vi "Select OPC Tags.vi"(7 "Mode":T1, 8 "error in":errorcluster, 11 "Section Ptr":T2 format="%.0x") -> (0 "error out":errorcluster)   [LabVIEW 2013, in "OPC UA Client System Explorer.lvlib"]
uses:
  OPC UA Client System Explorer.lvlib
  <vilib>/NI Veristand/Custom Device API/Custom Device Item Ref.ctl
  Types/Tag Selection Mode.ctl
  <vilib>/NI/AMC/Read Termination Message.vi
  <vilib>/NI/AMC/Create Single Message.vi
  <vilib>/NI/AMC/Update Message Routing Info.vi
  <vilib>/NI/AMC/Create Multiple Messages.vi
  <vilib>/NI/AMC/Globals.vi
  <vilib>/NI/AMC/Send Message.vi
  <vilib>/NI/AMC/AMC.lvlib
  <vilib>/NI Veristand/Custom Device API/Custom Device API.lvlib
panel:
  in  "OK":bool
  in  "Cancel":bool
  in  "Tree":string(tree)
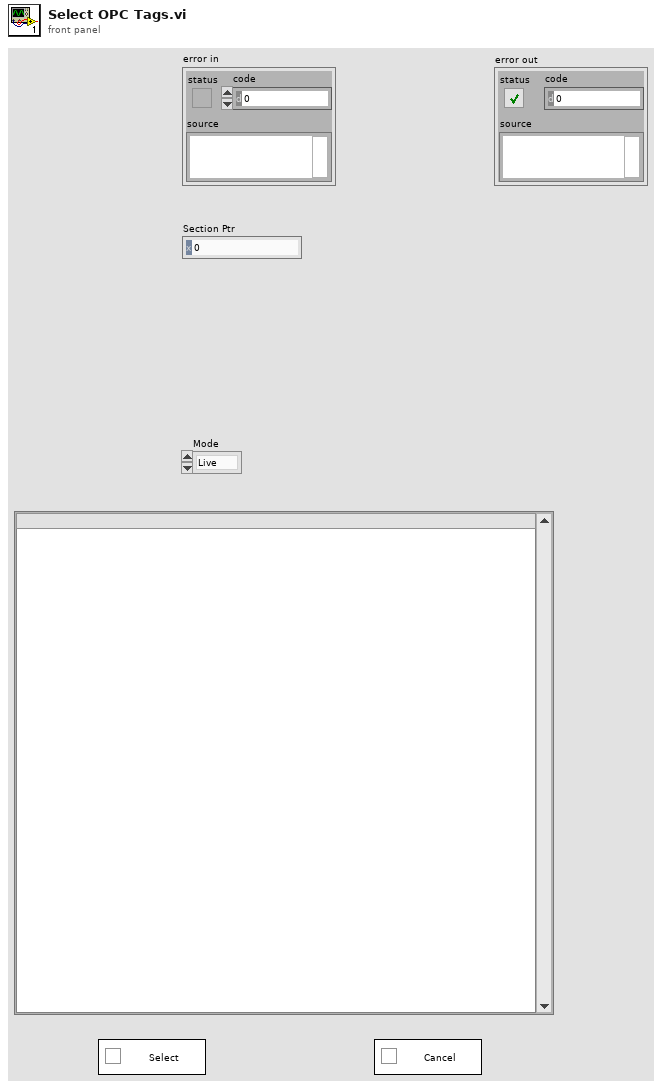
[diagram p1: front panel]
types:
  T1 = typedef "OPC UA Client System Explorer.lvlib/Tag Selection Mode.ctl" = enum8{"Live", "Offline"}
  T2 = typedef "Custom Device API.lvlib/Custom Device Item Ref.ctl" = u64
  T3 = cluster{"name":string, "node type":enum32{"Other", "Folder", "Item/Property"}, "DataType":u32, "access":enum16{"Null", "Read", "Write", "Read&Write"}, "description":string}
  T4 = typedef "AMC.lvlib/Message Queue.ctl" = refnum<queue>
  T5 = typedef "Custom Device API.lvlib/Custom Device Item Info.ctl" = cluster{"Name":string, "Is Channel":bool, "GUID":string, "Is Waveform":bool}
  T6 = typedef "OPC UA Client Shared.lvlib/Connection.Properties.ctl" = cluster{"Server IP Address":string, "Server Port":u16, "Message Mode":enum16{"None", "Sign", "Sign and Encrypt"}, "Security":enum16{"Basic256", "Basic128Rsa15"}, "User Name":string, "Password":string, "Client Certificate":path, "Server Certificate":path, "Server Certificate (RT)":path, "Client Certificate (RT)":path}
  T7 = typedef "LVPoint32TypeDef.ctl" = cluster{"Horizontal":i32, "Vertical":i32}
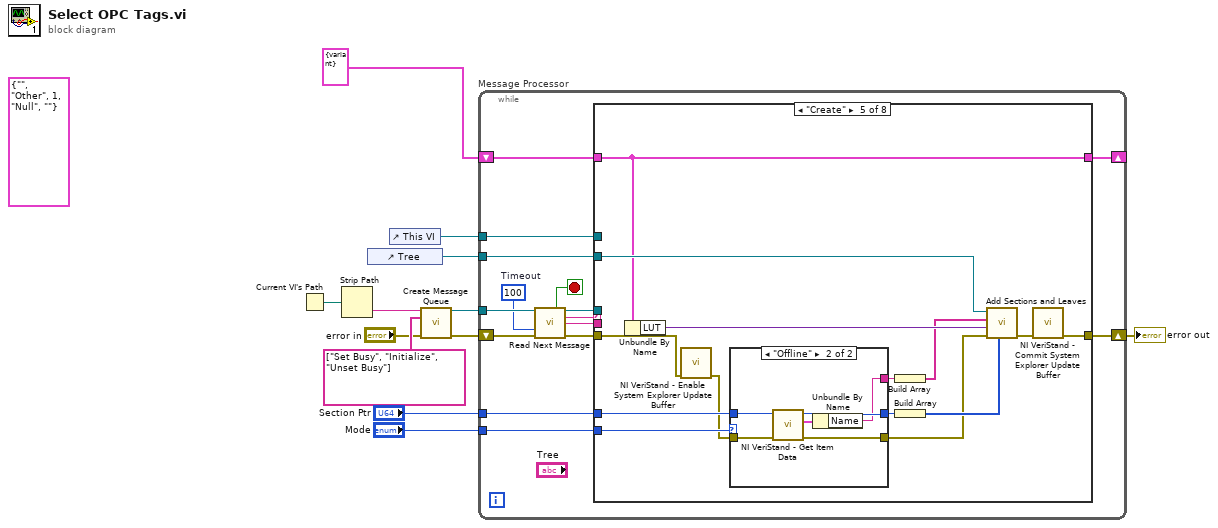
[diagram p0: block diagram]
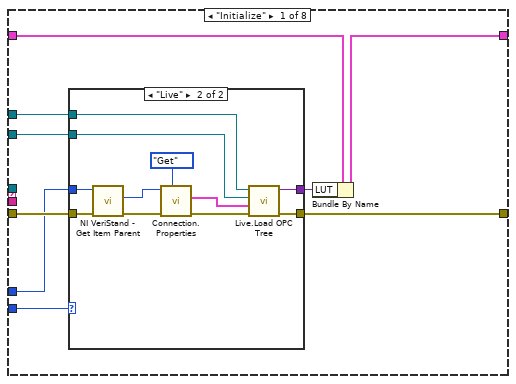
[diagram p2: hidden frame]
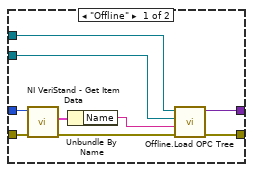
[diagram p3: hidden frame]
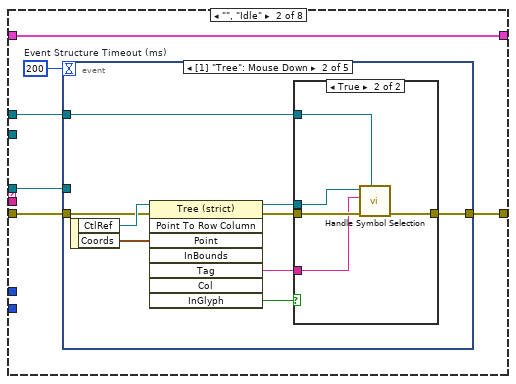
[diagram p4: hidden frame]
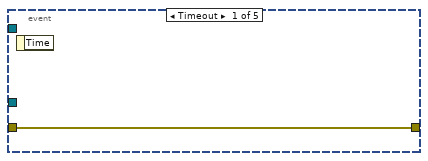
[diagram p5: hidden frame]
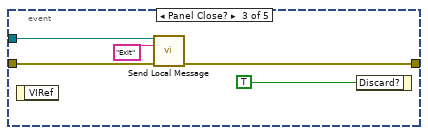
[diagram p7: hidden frame]
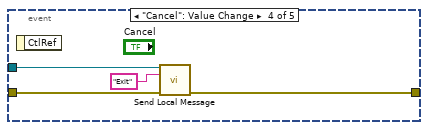
[diagram p8: hidden frame]
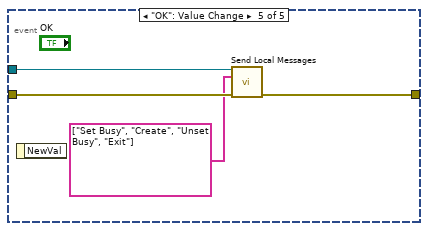
[diagram p9: hidden frame]
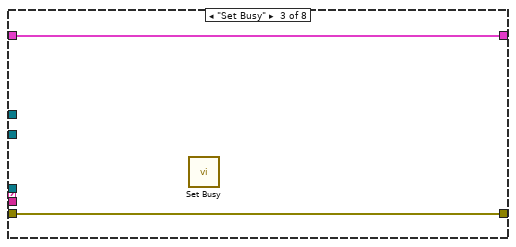
[diagram p10: hidden frame]
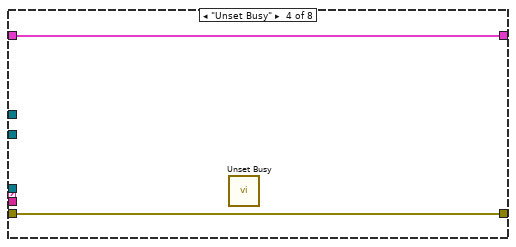
[diagram p11: hidden frame]
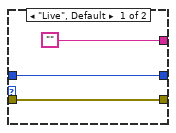
[diagram p12: hidden frame]
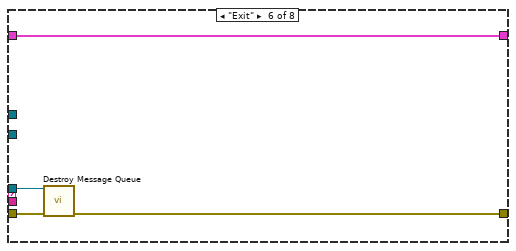
[diagram p13: hidden frame]
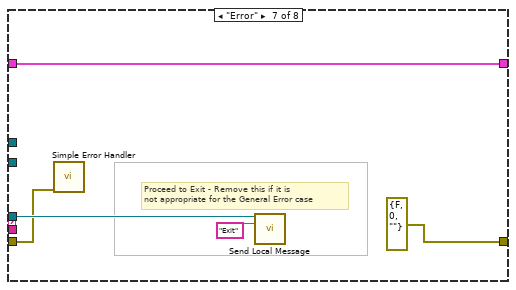
[diagram p14: hidden frame]
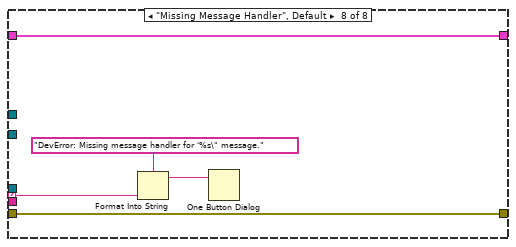
[diagram p15: hidden frame]
diagram:
  (unwired) T3 {"name"="", "node type"=enum."Other", "DataType"=1, "access"=enum."Null", "description"=""} ("node attribute")
  n1 = Current VI's Path() -> (path=w8:path)
  n2 = Strip Path(path=w8) -> (name=w11:string)  [unwired: 1 out]
  n3 = control-ref of="Tree"() -> (w5:refnum<vi>)
  n4 = control-ref of="This VI"() -> (w4:refnum<vi>)
  n5 = call <vilib>:"Create Message Queue.vi"("message queue name"=w11, "initial message names"=string[] ["Set Busy", "Initialize", "Unset Busy"], "error in"="error in") -> ("message queue out"=w10:T4, "error out"=w9:errorcluster)  [unwired: 11 in]
  n6 = while "Message Processor" {
    shift-left: w9 -> [w23]
    shift-right: [w27] -> w6
    tunnel: w10 -> [w24]
    tunnel: w5 -> [w18]
    tunnel: w4 -> [w17]
    shift-right: [w16] -> _
    shift-left: cluster{"LUT":variant} {"LUT"=variant} -> [w15]
    tunnel: "Section Ptr" -> [w14]
    tunnel: "Mode" -> [w13]
    stop <- w26 stop-if-true
    w19 = 100  # Timeout
    n7 = call <vilib>:"Read Next Message.vi"("message queue in"=w24, "timeout (1 ms)"=w19, "error in"=w23) -> ("exit process?"=w26:bool, "message queue out"=w25:T4, "message name"=w21:string, "message value"=w20:string, "error out"=w22:errorcluster)  [unwired: 5 in, 3 out]
    n8 = case shown="\"Create\"" w21 {
      selector: w21 -> [_ _ _ _ _ _ _ w131]
      tunnel: w25 -> [_ w61 _ _ _ w121 w126 _]
      tunnel: w22 -> [w31 w60 w92 w94 w104 w122 w124 w132]
      tunnel: [w36 w59 w92 w94 w102 w120 errorcluster {"status"=FALSE, "code"=0, "source"=""} ("error out") w132] -> w27
      tunnel: w20 -> [_ _ _ _ _ _ _ _]
      tunnel: w18 -> [w35 _ _ _ w109 _ _ _]
      tunnel: w17 -> [w34 w57 _ _ _ _ _ _]
      tunnel: [w32 w58 w93 w95 w107 w119 w123 w128] -> w16
      tunnel: w15 -> [w33 w58 w93 w95 w107 w119 w123 w128]
      tunnel: w14 -> [w30 _ _ _ w100 _ _ _]
      tunnel: w13 -> [w28 _ _ _ w101 _ _ _]
      frame "Initialize" {
        n9 = case shown="\"Live\"" w28 {
          tunnel: [w45 w56] -> w36
          tunnel: w35 -> [w44 w55]
          tunnel: w34 -> [w43 w54]
          tunnel: w31 -> [w39 w53]
          tunnel: w30 -> [w40 w52]
          tunnel: [w42 w50] -> w29
          frame "Offline" {
            n10 = call <vilib>:"NI VeriStand - Get Item Data.vi"("error in (no error)"=w39, "Item Ref in"=w40) -> ("error out"=w38:errorcluster, "Item Info"=w41:T5)  [unwired: 8 out]
            n11 = Unbundle By Name(w41) -> ("Name"=w37:string)
            n12 = call "Offline.Load OPC Tree.vi"("error in"=w38, "Channel"=w37, "Tree"=w44, "VI in"=w43) -> ("error out"=w45:errorcluster, "LUT"=w42:variant)  [unwired: 6 in]
          }
          frame "Live" {
            n13 = call <vilib>:"NI VeriStand - Get Item Parent.vi"("error in (no error)"=w53, "Item Ref in"=w52) -> ("error out"=w47:errorcluster, "Parent Ref"=w46:T2)  [unwired: 6 in, 2 out]
            n14 = call "Connection.Properties.vi"("Action"=enum8{"Get", "Set"}."Get", "error in (no error)"=w47, "Item Ref in"=w46) -> ("error out"=w51:errorcluster, "Connection.Properties"=w49:T6)  [unwired: 6 in, 1 out]
            n15 = call "Live.Load OPC Tree.vi"("error in (no error)"=w51, "Connection.Properties"=w49, "Tree"=w55, "VI in"=w54) -> ("error out"=w56:errorcluster, "LUT"=w50:variant)  [unwired: 6 in]
          }
        }
        n16 = Bundle By Name(cluster=w33, "LUT"=w29) -> (w32:cluster{"LUT":variant})
      }
      frame "", "Idle" {
        w62 = 200  # Event Structure Timeout (ms)
        n17 = event shown="[1] \"Tree\": Mouse Down" {
          selector: _ -> [_ _ _ _ _]
          dyn-events: _ -> [_ _ _ _ _]
          timeout: w62 -> [_ _ _ _ _]
          tunnel: w61 -> [_ _ w82 w86 w90]
          tunnel: w60 -> [w63 w70 w81 w84 w91]
          tunnel: [w63 w65 w80 w85 w89] -> w59
          tunnel: w57 -> [_ w64 _ _ _]
          event Timeout {
            n18 = event-data() -> ()  [unwired: 2 out]
          }
          event "Tree": Mouse Down {
            n19 = event-data() -> ("CtlRef"=w72:refnum<vi>, "Coords"=w71:T7)  [unwired: 1 out]
            n20 = invoke class="Tree (strict)" method="Point To Row Column"(reference=w72, error in=w70, "Point"=w71) -> (reference out=w66:refnum<vi>, error out=w68:errorcluster, "Tag"=w67:string, "InGlyph"=w69:bool)  [unwired: 5 in, 4 out]
            n21 = case shown="True" w69 {
              tunnel: w68 -> [w73 w78]
              tunnel: w67 -> [_ w76]
              tunnel: w66 -> [_ w77]
              tunnel: [w73 w75] -> w65
              tunnel: w64 -> [_ w74]
              frame False {
              }
              frame True {
                n22 = call "Handle Symbol Selection.vi"("This VI"=w74, "error in"=w78, "Tag"=w76, "CtlRef"=w77) -> ("error out"=w75:errorcluster)  [unwired: 7 in]
              }
            }
          }
          event Panel Close? {
            n23 = event-data() -> ()  [unwired: 2 out]
            n24 = call <vilib>:"Send Local Message.vi"("message queue in"=w82, "message name"="Exit", "error in"=w81) -> ("error out"=w80:errorcluster)  [unwired: 10 in, 2 out]
            n25 = event-data("Discard?"=TRUE) -> ()  [unwired: 1 in, 1 out]
          }
          event "Cancel": Value Change {
            n26 = event-data() -> ()  [unwired: 2 out]
            n27 = call <vilib>:"Send Local Message.vi"("message queue in"=w86, "message name"="Exit", "error in"=w84) -> ("error out"=w85:errorcluster)  [unwired: 10 in, 2 out]
          }
          event "OK": Value Change {
            n28 = event-data() -> ()  [unwired: 2 out]
            n29 = call <vilib>:"Send Local Messages.vi"("message queue in"=w90, "message names"=string[] ["Set Busy", "Create", "Unset Busy", "Exit"], "error in"=w91) -> ("error out"=w89:errorcluster)  [unwired: 10 in, 2 out]
          }
        }
      }
      frame "Set Busy" {
        n30 = call <vilib>:"Set Busy.vi"() -> ()  [unwired: 10 in, 2 out]
      }
      frame "Unset Busy" {
        n31 = call <vilib>:"Unset Busy.vi"() -> ()  [unwired: 11 in, 1 out]
      }
      frame "Create" {
        n32 = Unbundle By Name(w107) -> ("LUT"=w106:variant)
        n33 = call <vilib>:"NI VeriStand - Enable System Explorer Update Buffer.vi"("error in (no error)"=w104) -> ("error out"=w98:errorcluster)  [unwired: 10 in]
        n34 = case shown="\"Offline\"" w101 {
          tunnel: w100 -> [w112 w115]
          tunnel: [w112 w114] -> w99
          tunnel: w98 -> [w111 w117]
          tunnel: [w111 w116] -> w97
          tunnel: ["" w113] -> w96
          frame "Live", Default {
          }
          frame "Offline" {
            n35 = call <vilib>:"NI VeriStand - Get Item Data.vi"("error in (no error)"=w117, "Item Ref in"=w115) -> ("error out"=w116:errorcluster, "Item Info"=w118:T5, "Item Ref out"=w114:T2)  [unwired: 7 out]
            n36 = Unbundle By Name(w118) -> ("Name"=w113:string)
          }
        }
        n37 = Build Array(w96) -> (w105:string[])
        n38 = Build Array(w99) -> (w108:T2[])
        n39 = call "Add Sections and Leaves.vi"("VS Refs"=w108, "error in (no error)"=w97, "LUT"=w106, "Items"=w105, "TreeControl in"=w109) -> ("error out"=w103:errorcluster)  [unwired: 6 in]
        n40 = call <vilib>:"NI VeriStand - Commit System Explorer Update Buffer.vi"("error in (no error)"=w103) -> ("error out"=w102:errorcluster)  [unwired: 10 in]
      }
      frame "Exit" {
        n41 = call <vilib>:"Destroy Message Queue.vi"("message queue in"=w121, "error in"=w122) -> ("error out"=w120:errorcluster)  [unwired: 11 in, 2 out]
      }
      frame "Error" {
        # "Proceed to Exit - Remove this if it is\nnot appropriate for the General Error case"
        n42 = call <vilib>:"Simple Error Handler.vi"("error in (no error)"=w124) -> ()  [unwired: 1 in, 8 out]
        n43 = call <vilib>:"Send Local Message.vi"("message queue in"=w126, "message name"="Exit") -> ()  [unwired: 11 in, 3 out]
      }
      frame "Missing Message Handler", Default {
        n44 = Format Into String(format string="DevError: Missing message handler for '%s\" message." ("message"), w131) -> (resulting string=w129:string)  [unwired: 2 in, 1 out]
        n45 = One Button Dialog(message=w129) -> ()  [unwired: 2 out]
      }
    }
  }
  "error out" <- w6
